vi "scan_format_chart.vi"(8 "error in (no error)":errorcluster, 10 "info":T1, 11 "scan_panel in":refnum<class "scan_panel.lvclass">) -> (0 "error out":errorcluster, 3 "panel out":refnum<class "scan_panel.lvclass">)   [LabVIEW 2015, in "scan_panel.lvclass"]
uses:
  scan_panel.lvclass
  scan_hdf5_log/initialization_data.ctl
  <vilib>/Utility/miscctls.llb/LVOffsetAndMultiplierTypeDef.ctl
  UI/panel_class/panel.lvclass/panel.ctl
  UI/panel_class/panel.lvclass
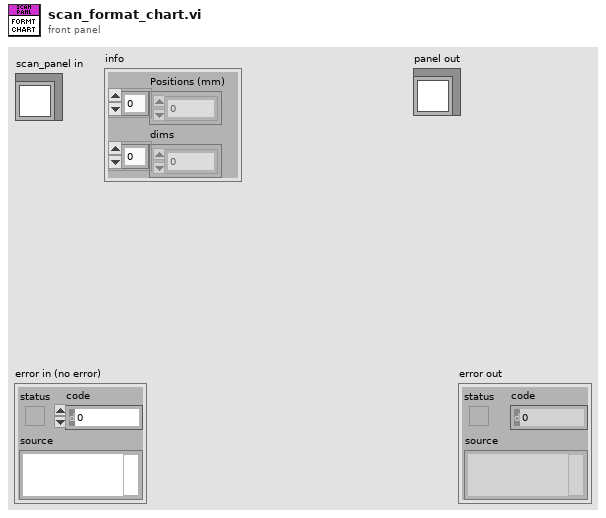
[diagram p1: front panel]
types:
  T1 = typedef "initialization_data.ctl" = cluster{"Positions (mm)":dbl[], "dims":u32[]}
  T2 = cluster{dbl, dbl, dbl, dbl, dbl, dbl, dbl, dbl}[]
  T3 = typedef "LVOffsetAndMultiplierTypeDef.ctl" = cluster{"Offset":dbl, "Multiplier":dbl}
  T4 = typedef "ui_plot_references.ctl" = cluster{"plots":refnum<vi>, "chart":refnum<vi>, "graph":refnum<vi>, "map":refnum<vi>, "XY Graph":refnum<vi>}
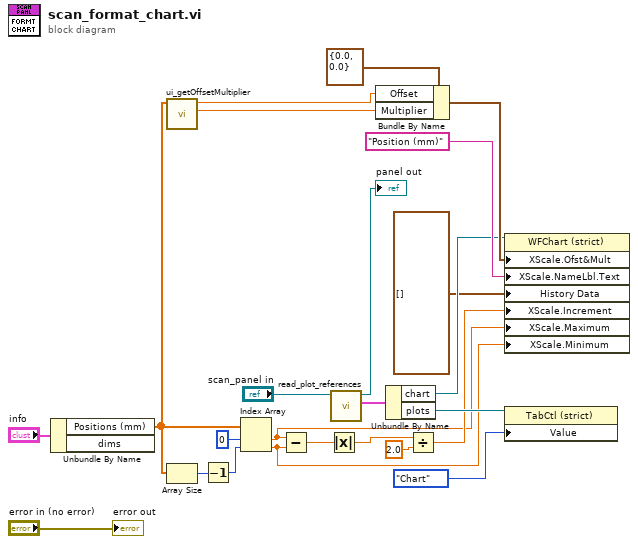
[diagram p0: block diagram]
diagram:
  n1 = Unbundle By Name("info") -> ("Positions (mm)"=w12:dbl[])  [unwired: 1 out]
  n2 = call "ui_getOffsetMultiplier.vi"("Axis"=w12) -> ("Multiplier"=w16:dbl, "Offset"=w17:dbl)  [unwired: 9 in]
  n3 = Array Size(array=w12) -> (size(s)=w4:i32)
  n4 = Decrement(x=w4) -> (x-1=w10:i32)
  n5 = Index Array(array=w12, index #1=0 ("index"), index #2=w10) -> (element #1=w3:dbl, element #2=w2:dbl)
  n6 = Subtract(x=w3, y=w2) -> (x-y=w9:dbl)
  n7 = Absolute Value(x=w9) -> (abs(x)=w8:dbl)
  n8 = call "read_plot_references.vi"("panel in"="scan_panel in") -> ("plot_references"=w21:T4, "panel out"=→"panel out":refnum<class "scan_panel.lvclass">)  [unwired: 8 in, 1 out]
  n9 = Bundle By Name(cluster=T3 {"Offset"=0.0, "Multiplier"=0.0} ("X Scale.Offset and Multiplier"), "Offset"=w17, "Multiplier"=w16) -> (w14:T3)
  n10 = Unbundle By Name(w21) -> ("chart"=w13:refnum<vi>, "plots"=w22:refnum<vi>)
  n11 = Divide(x=w8, y=2.0) -> (x/y=w6:dbl)
  n12 = property class="WFChart (strict)"(reference=w13, "XScale.Ofst&Mult"=w14, "XScale.NameLbl.Text"="Position (mm)" ("Y Scale.Name Label.Text"), "History Data"=T2 [], "XScale.Increment"=w6, "XScale.Maximum"=w3, "XScale.Minimum"=w2) -> ()  [unwired: 1 in, 2 out]
  n13 = property class="TabCtl (strict)"(reference=w22, "Value"=enum32{"Chart", "Graph", "Map", "XY Graph"}."Chart") -> ()  [unwired: 1 in, 2 out]
  "error out" <- "error in (no error)"
